vi "Export Report.vi"(8 "error in (no error)":errorcluster, 10 "Storage":refnum<class "Test Event Storage.lvclass">, 11 "Basic Test Manager in":refnum<class "Basic Test Manager.lvclass">) -> (0 "error out":errorcluster, 3 "Basic Test Manager out":refnum<class "Basic Test Manager.lvclass">)   [LabVIEW 2020, in "Caraya.lvlib" / "Basic Test Manager.lvclass"]
uses:
  Basic Test Manager.lvclass
  Test Event Storage/Test Event Storage.lvclass
  Test Report/Test Report.lvclass
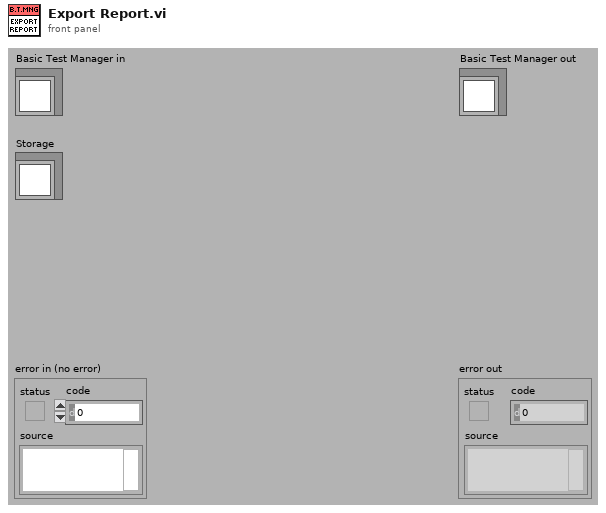
[diagram p1: front panel]
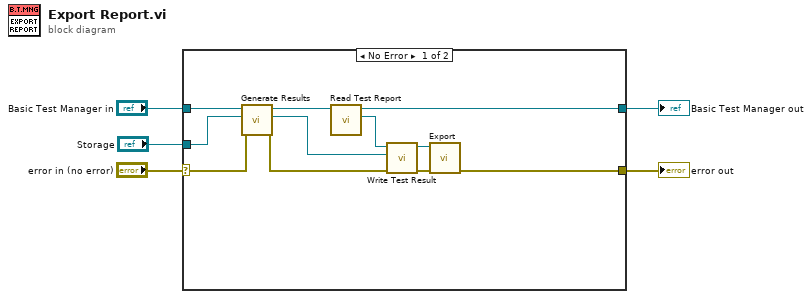
[diagram p0: block diagram]
diagram:
  n1 = case shown="No Error" "error in (no error)" {
    selector: "error in (no error)" -> [w11 w18]
    tunnel: [w16 w18] -> w4
    tunnel: [w15 w17] -> w2
    tunnel: "Basic Test Manager in" -> [w13 w17]
    tunnel: "Storage" -> [w14 _]
    frame No Error {
      n2 = call "Generate Results.vi"("error in (no error)"=w11, "Storage"=w14, "Basic Test Manager in"=w13) -> ("error out"=w8:errorcluster, "Test Result"=w6:refnum<class "Test Result.lvclass">, "Basic Test Manager out"=w12:refnum<class "Basic Test Manager.lvclass">)  [unwired: 6 in]
      n3 = call "Read Test Report.vi"("Basic Test Manager"=w12) -> ("Test Report"=w10:refnum<class "Test Report.lvclass">, "Basic Test Manager"=w15:refnum<class "Basic Test Manager.lvclass">)  [unwired: 9 in]
      n4 = call "Write Test Result.vi"("error in (no error)"=w8, "Test Result"=w6, "Test Report in"=w10) -> ("error out"=w7:errorcluster, "Test Report out"=w9:refnum<class "Test Report.lvclass">)  [unwired: 7 in]
      n5 = call-dynamic "Export.vi"("error in (no error)"=w7, "Test Report in"=w9) -> ("error out"=w16:errorcluster)  [unwired: 8 in, 1 out]
    }
    frame Error {
    }
  }
  "error out" <- w4
  "Basic Test Manager out" <- w2
